vi "8_ProgrammingTests.vi"() -> ()   [LabVIEW 2012]
uses:
  <userlib>/BotSpeak/VIs/Scripting/URAPI_ForStart_num.vi
  <userlib>/BotSpeak/VIs/Scripting/URAPI_WriteDigitalOut.vi
  <userlib>/BotSpeak/VIs/Scripting/URAPI_ReadDigitalIn.vi
  <userlib>/BotSpeak/VIs/Scripting/URAPI_InitTimer_num.vi
  <userlib>/BotSpeak/VIs/Scripting/URAPI_SetPWM_num.vi
  <userlib>/BotSpeak/VIs/Scripting/URAPI_Delay_num.vi
  <userlib>/BotSpeak/VIs/Scripting/URAPI_Timer_num.vi
panel:
  out "BotSpeak":string="SET var2,0\nSET var,0\nSCRIPT\nSET count0,0\nSET DIO[count0],1\nSET variable,DIO[count0]\nADD var,variable\nADD count0,1\nIF (count0 < 14) GOTO 3\nSET count2,0\nSET DIO[count2],0\nSET variable,DIO[count2]\nADD var2,variable\nADD count2,1\nIF (count2 < 14) GOTO 10\nSET TMR[0],0\nSET timer,0\nSET count4,0\nIF ~(timer < 100) GOTO 34\nSET PWM[50],0\nGOTO 24\nWAIT 1.000000\nIF ~(var > var2) GOTO 28\nSET ans,1\nGOTO 30\nSET ans,0\nSET timer,TMR[0]\nADD count4,1\nGOTO 19\nend\nENDSCRIPT\nRUN&WAIT 0\nGET var\nGET var2\nGET ans\n"
  out "expected response":string="0\r\nstart script\r\nend script\r\n......................................................................................................................................................................................................................................................\nDone\r\n14\r\n1\r\n1\r\n"
  out "response":string="0\r\nstart script\r\nend script\r\n......................................................................................................................................................................................................................................................\nDone\r\n14\r\n1\r\n1\r\n"
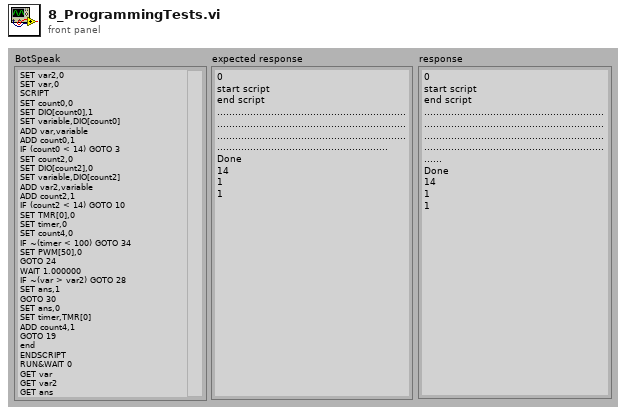
[diagram p1: front panel]
types:
  T1 = typedef "URAPI_Control.ctl" = cluster{"Script":string, "Whiles":u8[], "Ifs":u8[], "Supress Err":bool, "Errors":string}
  T2 = typedef "BotSpeak_Control.ctl" = cluster{"Address":string, "Reply EOF":string, "Hardware":path, "Retries":i8, "Timeout":i32}
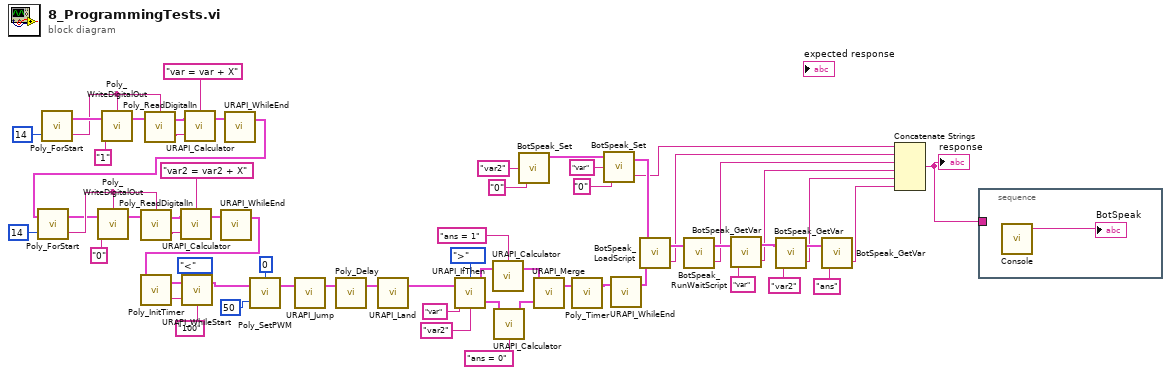
[diagram p0: block diagram]
diagram:
  n1 = call-poly <userlib>:"Poly_ForStart.vi"("Iterations"=u16 14) -> ("variable"=w39:string, "URAPI Script Out"=w43:T1)  [unwired: 3 in]
  n2 = call-poly <userlib>:"Poly_WriteDigitalOut.vi"("Variable In"="1", "URAPI Script"=w43, "Channel"=w39) -> ("URAPI Script"=w47:T1)  [unwired: 1 in, 1 out]
  n3 = call-poly <userlib>:"Poly_ReadDigitalIn.vi"("URAPI Script"=w47, "Channel"=w39) -> ("Variable Out"=w36:string, "URAPI Script"=w37:T1)  [unwired: 2 in]
  n4 = call <userlib>:"URAPI_Calculator.vi"("X"=w36, "URAPI Script"=w37, "Formula"="var = var + X") -> ("URAPI Script"=w38:T1)  [unwired: 1 in, 1 out]
  n5 = call <userlib>:"URAPI_WhileEnd.vi"("URAPI Script"=w38) -> ("URAPI Script Out"=w25:T1)  [unwired: 4 in]
  n6 = call-poly <userlib>:"Poly_ForStart.vi"("Iterations"=u16 14, "URAPI Script"=w25) -> ("variable"=w30:string, "URAPI Script Out"=w27:T1)  [unwired: 2 in]
  n7 = call-poly <userlib>:"Poly_WriteDigitalOut.vi"("Variable In"="0", "URAPI Script"=w27, "Channel"=w30) -> ("URAPI Script"=w26:T1)  [unwired: 1 in, 1 out]
  n8 = call-poly <userlib>:"Poly_ReadDigitalIn.vi"("URAPI Script"=w26, "Channel"=w30) -> ("Variable Out"=w33:string, "URAPI Script"=w32:T1)  [unwired: 2 in]
  n9 = call <userlib>:"URAPI_Calculator.vi"("X"=w33, "URAPI Script"=w32, "Formula"="var2 = var2 + X") -> ("URAPI Script"=w31:T1)  [unwired: 1 in, 1 out]
  n10 = call <userlib>:"URAPI_WhileEnd.vi"("URAPI Script"=w31) -> ("URAPI Script Out"=w9:T1)  [unwired: 4 in]
  n11 = call-poly <userlib>:"Poly_InitTimer.vi"("URAPI Script"=w9) -> ("Variable out"=w11:string, "URAPI Script out"=w10:T1)  [unwired: 3 in]
  n12 = call <userlib>:"URAPI_WhileStart.vi"("Variable In"=w11, "Compare to"="100", "URAPI Script"=w10, "Comparison"=enum16{">", "<", "=", "!="}."<") -> ("URAPI Script Out"=w6:T1)  [unwired: 1 out]
  n13 = call-poly <userlib>:"Poly_SetPWM.vi"("Variable In"=u8 50, "URAPI Script"=w6, "Port"=u8 0) -> ("URAPI Script"=w46:T1)  [unwired: 1 in, 1 out]
  n14 = call <userlib>:"URAPI_Jump.vi"("URAPI Script"=w46) -> ("URAPI Script"=w45:T1)  [unwired: 4 in]
  n15 = call-poly <userlib>:"Poly_Delay.vi"("URAPI Script"=w45) -> ("URAPI Script out"=w44:T1)  [unwired: 4 in]
  n16 = call <userlib>:"URAPI_Land.vi"("URAPI Script"=w44) -> ("URAPI Script Out"=w42:T1)  [unwired: 4 in]
  n17 = call <userlib>:"URAPI_IfThen.vi"("Variable In"="var", "Compare to"="var2", "URAPI Script"=w42, "Comparison"=enum16{">", "<", "=", "!="}.">") -> ("URAPI False"=w16:T1, "URAPI True"=w19:T1)
  n18 = call <userlib>:"URAPI_Calculator.vi"("URAPI Script"=w19, "Formula"="ans = 1") -> ("URAPI Script"=w18:T1)  [unwired: 2 in, 1 out]
  n19 = call <userlib>:"URAPI_Calculator.vi"("URAPI Script"=w16, "Formula"="ans = 0") -> ("URAPI Script"=w15:T1)  [unwired: 2 in, 1 out]
  n20 = call <userlib>:"BotSpeak_Set.vi"("value"="0", "Variable In"="var2") -> ("Bot Settings"=w1:T2)  [unwired: 1 in, 1 out]
  n21 = call <userlib>:"URAPI_Merge.vi"("URAPI False"=w15, "URAPI True"=w18) -> ("URAPI Script"=w5:T1)  [unwired: 3 in]
  n22 = call-poly <userlib>:"Poly_Timer.vi"("URAPI Script"=w5) -> ("URAPI Script out"=w4:T1)  [unwired: 3 in, 1 out]
  n23 = call <userlib>:"BotSpeak_Set.vi"("value"="0", "Variable In"="var", "Bot Settings"=w1) -> ("response"=w48:string, "Bot Settings"=w49:T2)
  n24 = call <userlib>:"URAPI_WhileEnd.vi"("URAPI Script"=w4) -> ("URAPI Script Out"=w13:T1)  [unwired: 4 in]
  n25 = call <userlib>:"BotSpeak_LoadScript.vi"("URAPI Script"=w13, "Bot Settings"=w49) -> ("total response"=w55:string, "Bot Settings"=w61:T2)
  n26 = call <userlib>:"BotSpeak_RunWaitScript.vi"("Bot Settings"=w61) -> ("response"=w54:string, "Bot Settings"=w60:T2)  [unwired: 1 in]
  n27 = call <userlib>:"BotSpeak_GetVar.vi"("Variable In"="var", "Bot Settings"=w60) -> ("value"=w53:string, "Bot Settings out"=w57:T2)
  n28 = call <userlib>:"BotSpeak_GetVar.vi"("Variable In"="var2", "Bot Settings"=w57) -> ("value"=w52:string, "Bot Settings out"=w56:T2)
  n29 = call <userlib>:"BotSpeak_GetVar.vi"("Variable In"="ans" ("Formula"), "Bot Settings"=w56) -> ("value"=w51:string)  [unwired: 1 out]
  n30 = Concatenate Strings(w48, w55, w54, w53, w52, w51) -> (w50:string)
  "response" <- w50
  n31 = stacked-sequence {
    tunnel: w50 -> [_]
    frame #0 {
      n32 = call <userlib>:"Console.vi"() -> ("BotSpeak"=→"BotSpeak":string)  [unwired: 4 in, 1 out]
    }
  }
